vi "ParseDataMsg.vi"(8 "error in (no error)":errorcluster, 10 "JSON<>":string, 11 "DownStreamMsgHandler in":refnum<class "DownStreamMsgHandler.lvclass">) -> (0 "error out":errorcluster, 3 "DownStreamMsgHandler out":refnum<class "DownStreamMsgHandler.lvclass">)   [LabVIEW 2020, in "DownstreamMsgHandler.lvlib" / "DownStreamMsgHandler.lvclass"]
uses:
  DownStreamMsgHandler.lvclass
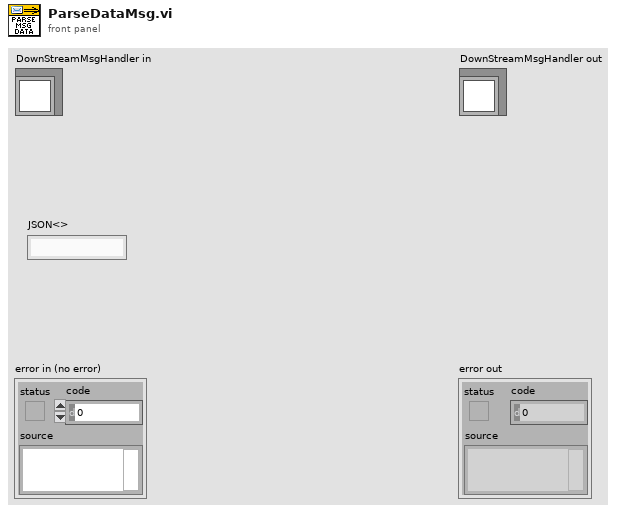
[diagram p1: front panel]
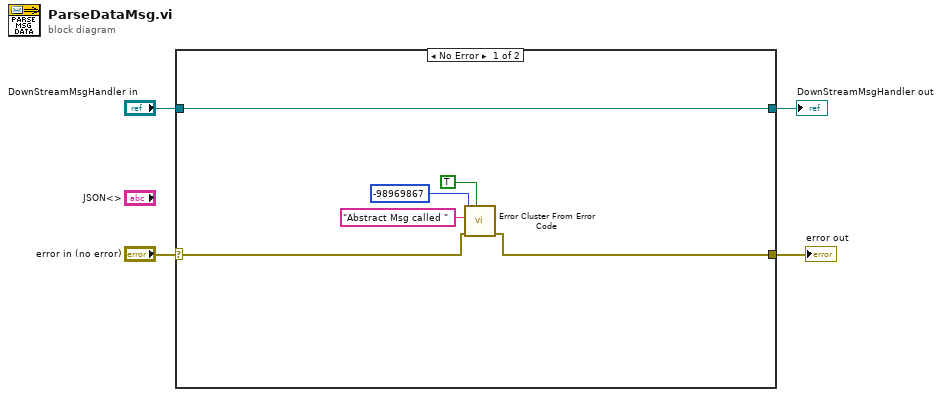
[diagram p0: block diagram]
diagram:
  n1 = case shown="No Error" "error in (no error)" {
    selector: "error in (no error)" -> [w9 w12]
    tunnel: [w8 w12] -> w3
    tunnel: [w10 w11] -> w1
    tunnel: "DownStreamMsgHandler in" -> [w10 w11]
    frame No Error {
      n2 = call <vilib>:"Error Cluster From Error Code.vi"("show call chain? (False)"=TRUE, "error in (no error)"=w9, "error message (\"\")"="Abstract Msg called " ("error message (\"\")"), "error code (0)"=-98969867) -> ("error out"=w8:errorcluster)  [unwired: 5 in]
    }
    frame Error {
    }
  }
  "error out" <- w3
  "DownStreamMsgHandler out" <- w1
